vi "Translator DLL InputOutput.vi"(0 "Input":variant=variant("Function Name"=variant(string "Strip Path"), "Input Datatypes"=variant(string[] ["error", "int"]), "Inputs"=variant(string[] ["error in", "x"]), "Node refnum"=variant(refnum<vi> refnum), "Output Datatypes"=variant(string[] ["int"]), "Outputs"=variant(string[] ["a"])), 11 "error in (no error)":errorcluster) -> (4 "Output":variant=variant("Defines"=variant(string[] []), "Includes"=variant(string[] []), "Replaced Code"=variant(string "/* LabVIEW system function 'Strip Path' not found. */")), 15 "error out":errorcluster)   [LabVIEW 2014, in "DLL InputOutput Lib.lvlib"]
doc: "source: https://www.arduino.cc/en/Reference/SPIEnd\n\nDisables the SPI bus (leaving pin modes unchanged).\n\nSyntax\n SPI.end()\n\nParameters\n None\n\nReturns\n None"
uses:
  DLL InputOutput Lib.lvlib
panel:
  out "Outputs":string[](array[string])
  out "Inputs":string[](array[string])
  out "Output Datatypes":string[](array[string])
  out "Input Datatypes":string[](array[string])
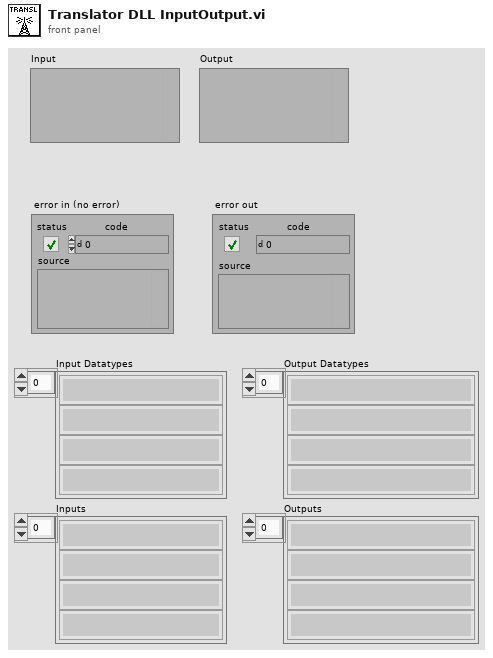
[diagram p1: front panel]
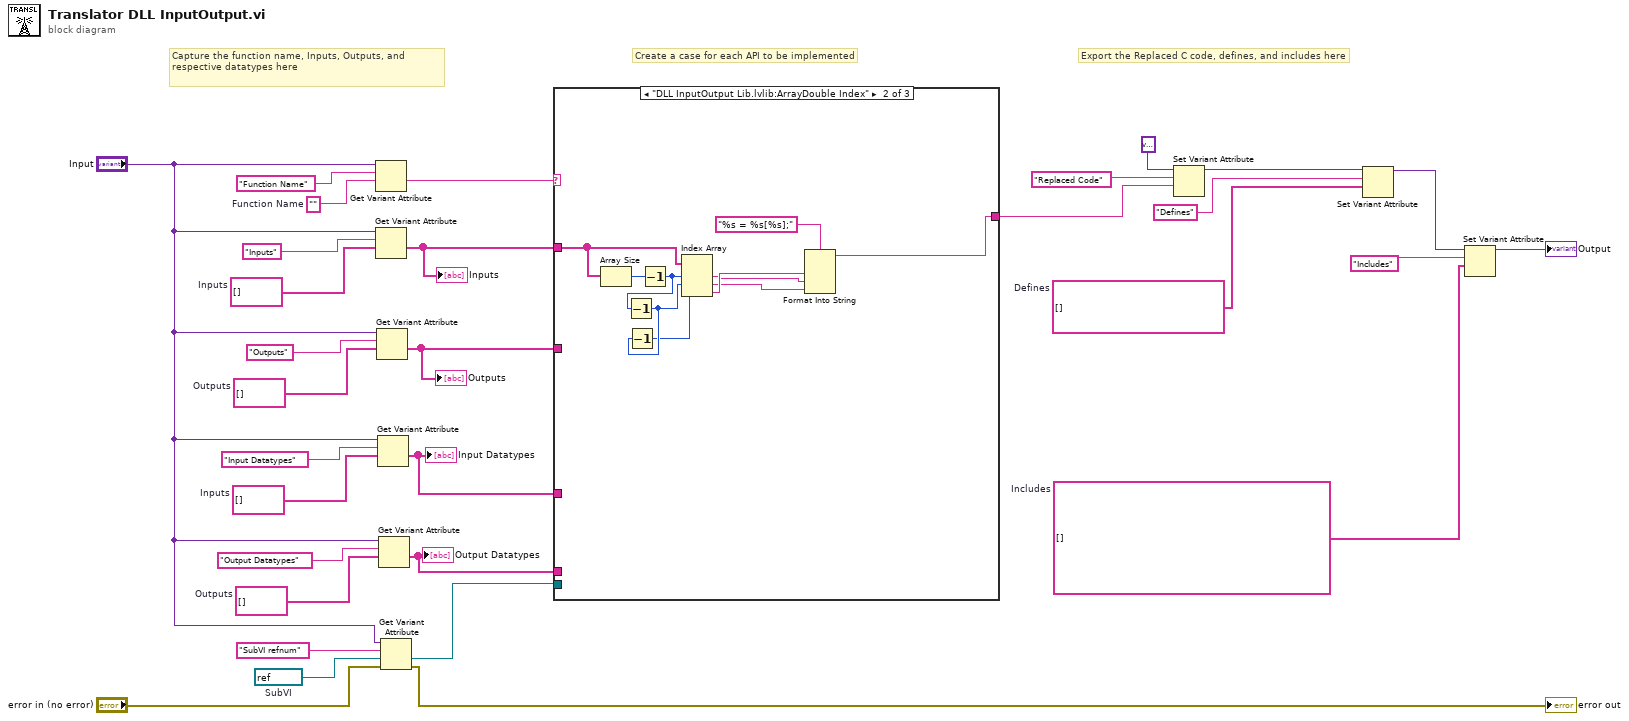
[diagram p0: block diagram]
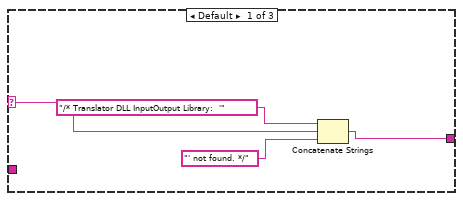
[diagram p2: hidden frame]
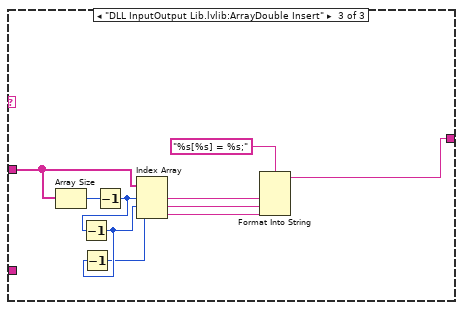
[diagram p3: hidden frame]
diagram:
  w7 = refnum<vi> refnum  # SubVI
  w4 = string[] []  # Defines
  w17 = string[] []  # Outputs
  w18 = string[] []  # Inputs
  w3 = string[] []  # Includes
  w27 = string[] []  # Outputs
  w28 = string[] []  # Inputs
  w29 = ""  # Function Name
  # "Capture the function name, Inputs, Outputs, and respective datatypes here"
  # "Export the Replaced C code, defines, and includes here"
  # "Create a case for each API to be implemented"
  n1 = Get Variant Attribute(Variant="Input", name="Function Name", default value (empty Variant)=w29) -> (value=w24:string)  [unwired: 1 in, 3 out]
  n2 = Get Variant Attribute(Variant="Input", name="Inputs", default value (empty Variant)=w28) -> (value=w14:string[])  [unwired: 1 in, 3 out]
  "Inputs" <- w14
  n3 = Get Variant Attribute(Variant="Input", name="Outputs", default value (empty Variant)=w27) -> (value=w15:string[])  [unwired: 1 in, 3 out]
  "Outputs" <- w15
  n4 = Get Variant Attribute(Variant="Input", name="Input Datatypes", default value (empty Variant)=w18) -> (value=w10:string[])  [unwired: 1 in, 3 out]
  "Input Datatypes" <- w10
  n5 = Get Variant Attribute(Variant="Input", name="Output Datatypes", default value (empty Variant)=w17) -> (value=w5:string[])  [unwired: 1 in, 3 out]
  "Output Datatypes" <- w5
  n6 = Get Variant Attribute(Variant="Input", name="SubVI refnum", default value (empty Variant)=w7, error in="error in (no error)") -> (value=w6:refnum<vi>, error out=→"error out":errorcluster)  [unwired: 2 out]
  n7 = case shown="\"DLL InputOutput Lib.lvlib:ArrayDouble Index\"" w24 {
    selector: w24 -> [w34 _ _]
    tunnel: [w32 w39 w46] -> w23
    tunnel: w14 -> [_ w44 w54]
    tunnel: w15 -> [_ _ _]
    tunnel: w10 -> [_ _ _]
    tunnel: w6 -> [_ _ _]
    tunnel: w5 -> [_ _ _]
    frame Default {
      n8 = Concatenate Strings("/* Translator DLL InputOutput Library:  '", w34, "' not found. */") -> (w32:string)
    }
    frame "DLL InputOutput Lib.lvlib:ArrayDouble Index" {
      n9 = Array Size(array=w44) -> (size(s)=w45:i32)
      n10 = Decrement(x=w45) -> (x-1=w43:i32)
      n11 = Decrement(x=w43) -> (x-1=w41:i32)
      n12 = Decrement(x=w41) -> (x-1=w40:i32)
      n13 = Index Array(array=w44, index #1=w43, index #2=w41, index #3=w40) -> (element #1=w37:string, element #2=w36:string, element #3=w38:string)
      n14 = Format Into String(format string="%s = %s[%s];", w38, w37, w36) -> (resulting string=w39:string)  [unwired: 2 in, 1 out]
    }
    frame "DLL InputOutput Lib.lvlib:ArrayDouble Insert" {
      n15 = Array Size(array=w54) -> (size(s)=w55:i32)
      n16 = Decrement(x=w55) -> (x-1=w53:i32)
      n17 = Decrement(x=w53) -> (x-1=w49:i32)
      n18 = Decrement(x=w49) -> (x-1=w48:i32)
      n19 = Index Array(array=w54, index #1=w53, index #2=w49, index #3=w48) -> (element #1=w51:string, element #2=w50:string, element #3=w47:string)
      n20 = Format Into String(format string="%s[%s] = %s;", w51, w50, w47) -> (resulting string=w46:string)  [unwired: 2 in, 1 out]
    }
  }
  n21 = Set Variant Attribute(Variant=variant ("variant"), name="Replaced Code", value=w23) -> (Variant out=w13:variant)  [unwired: 1 in, 2 out]
  n22 = Set Variant Attribute(Variant=w13, name="Defines", value=w4) -> (Variant out=w12:variant)  [unwired: 1 in, 2 out]
  n23 = Set Variant Attribute(Variant=w12, name="Includes", value=w3) -> (Variant out=→"Output":variant)  [unwired: 1 in, 2 out]
